vi "Desplegar arreglos boleanos.vi"(8 "error in (no error)":errorcluster, 10 "Expected Response out":string, 11 "NXP in":refnum<class "NXP.lvclass">) -> (0 "error out":errorcluster, 1 "Puerto":string, 2 "output array":bool[](array[boolean]), 3 "NXP out":refnum<class "NXP.lvclass">)   [LabVIEW 2020, in "NXP.lvclass"]
uses:
  NXP.lvclass
  Abstract/Serial Device/Serial Device.lvclass
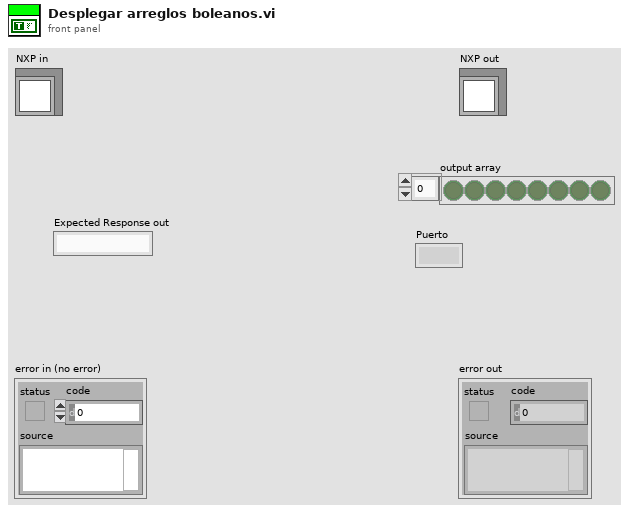
[diagram p1: front panel]
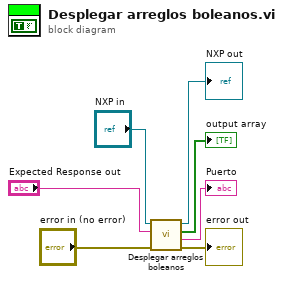
[diagram p0: block diagram]
diagram:
  n1 = call-parent "Desplegar arreglos boleanos.vi"("error in (no error)"="error in (no error)", "Expected Response out"="Expected Response out", "Serial Device in"="NXP in") -> ("error out"=→"error out":errorcluster, "Puerto"=→"Puerto":string, "output array"=→"output array":bool[], "Serial Device out"=→"NXP out":refnum<class "NXP.lvclass">)  [unwired: 5 in]
